vi "N58_Flask_Kill_timer.vi"(1 "DUTin":string) -> ()   [LabVIEW 2024, in "Neoway_flashing.lvlib"]
uses:
  Neoway_flashing.lvlib
  Launcher/SubVI/Global 1.vi
  Launcher/Launcher_DTU.lvlib
panel:
  out "DUT":string
  in  "String":string="N58 FLASHING"
  out "output":string
  out "Timer":u32
  in  "stop":bool
  in  "Loading symbol":u16(ring)
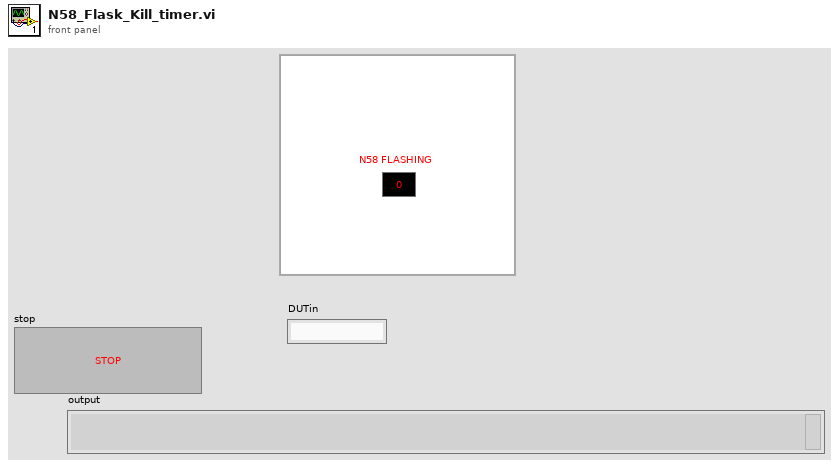
[diagram p1: front panel]
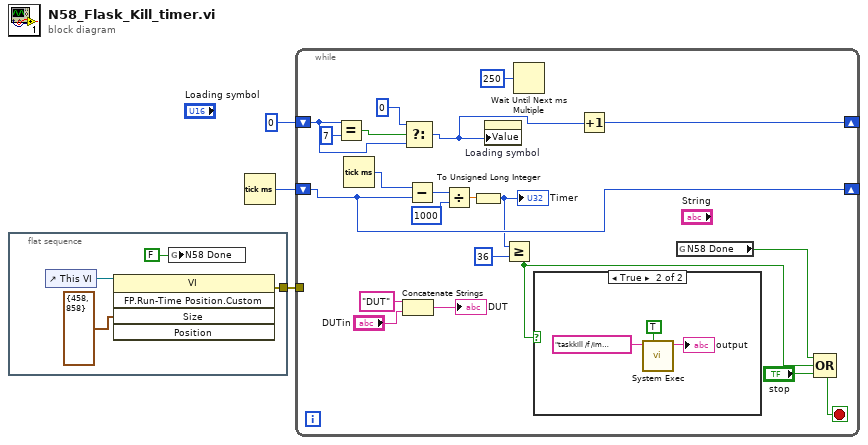
[diagram p0: block diagram]
diagram:
  n1 = flat-sequence {
    tunnel: [w6] -> w1
    frame #0 {
      n2 = control-ref of="This VI"() -> (w7:refnum<vi>)
      n3 = invoke class="VI" method="FP.Run-Time Position.Custom"(reference=w7, "Size"=cluster{"Top":i16, "Left":i16} {"Top"=458, "Left"=858} ("Position")) -> (error out=w6:errorcluster)  [unwired: 3 in, 4 out]
      n4 = global write "Global 1.vi" "N58 Done"(FALSE ("N58 Done")) -> ()
    }
  }
  n5 = Tick Count (ms)() -> (millisecond timer value=w2:u32)
  n6 = while {
    shift-right: [w22] -> _
    shift-left: u16 0 -> [w24]
    shift-right: [w17] -> _
    shift-left: w2 -> [w17]
    tunnel: w1 -> [_]
    stop <- w14 stop-if-true
    n7 = Equal?(x=w24, y=u16 7) -> (x = y?=w26:bool)
    n8 = Tick Count (ms)() -> (millisecond timer value=w21:u32)
    n9 = Concatenate Strings("DUT", "DUTin") -> (→"DUT":string)
    n10 = Select(t=u16 0 ("Loading symbol"), s=w26, f=w24) -> (s? t:f=w23:u16)
    n11 = Subtract(x=w21, y=w17) -> (x-y=w20:u32)
    n12 = Divide(x=w20, y=u32 1000) -> (x/y=w18:dbl)
    n13 = To Unsigned Long Integer(number=w18) -> (unsigned 32bit integer=w16:u32)
    "Timer" <- w16
    n14 = property on="Loading symbol" class="Ring (strict)"("Value"=w23) -> ()  [unwired: 2 in, 2 out]
    n15 = Greater Or Equal?(x=w16, y=u32 36) -> (x >= y?=w12:bool)
    n16 = Wait Until Next ms Multiple(millisecond multiple=u32 250) -> ()  [unwired: 1 out]
    n17 = case shown="True" w12 {
      frame False {
      }
      frame True {
        n18 = call <vilib>:"System Exec.vi"("wait until completion? (T)"=TRUE, "command line"="taskkill /f /im CmdDloader.exe") -> ("standard output"=→"output":string)  [unwired: 6 in, 3 out]
      }
    }
    n19 = Increment(x=w23) -> (x+1=w22:u16)
    n20 = global read "Global 1.vi" "N58 Done"() -> (w8:bool)
    n21 = Compound Arithmetic op=OR(w8, w12, "stop") -> (w14:bool)
  }
